vi "V7310.Job.Get.vi"(6 "timeout ms (5000)":i32=5000, 8 "error in":errorcluster, 11 "Connection in":refnum<k5>) -> (0 "error out":errorcluster, 2 "Job":string, 3 "Connection out":refnum<k5>)   [LabVIEW 2016]
uses:
  LowLevel/V7310.Commands.ctl
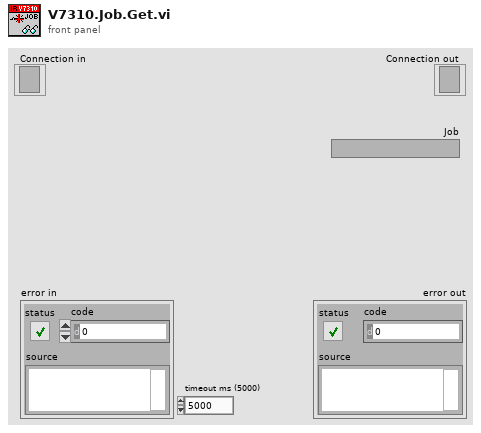
[diagram p1: front panel]
types:
  T1 = typedef "V7310.Commands.ctl" = enum16{"Start", "Stop", "GetStatus", "GetVarNames", "GetJobNames", "SetJob", "GetJob", "SetVars", "GetVars", "SetLayoutPosition", "SetRotation", "GetMessageID", "GetMessages", "ConfirmMessages", "DeleteMessages", "SetRTC", "GetRTC", "SetVarPosition", "SetIntensity", "GetIntensity", "SetStartTriggerDelay", "GetStartTriggerDelay", "SetStopTriggerDelay", "GetStopTriggerDelay", "SetConsecutiveTriggerDelay", "GetConsecutiveTriggerDelay", "SetMarkSpeed", "GetMarkSpeed"}
  T2 = typedef "V7310.ErrorLevels.ctl" = enum16{"OK", "Warning", "Error"}
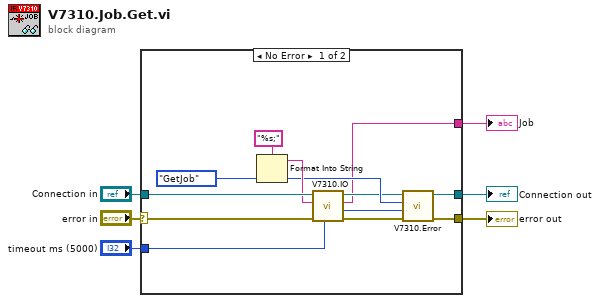
[diagram p0: block diagram]
diagram:
  n1 = case shown="No Error" "error in" {
    selector: "error in" -> [w16 w18]
    tunnel: "Connection in" -> [w17 w19]
    tunnel: [w8 w19] -> w5
    tunnel: "timeout ms (5000)" -> [w10 _]
    tunnel: [w9 w18] -> w2
    tunnel: [w7 _] -> w1
    frame No Error {
      w13 = V7310.Commands."GetJob" ("Cmd")
      n2 = Format Into String(format string="%s;", w13) -> (resulting string=w14:string)  [unwired: 2 in, 1 out]
      n3 = call "V7310.IO.vi"("timeout ms (5000)"=w10, "error in"=w16, "Data in"=w14, "Connection in"=w17) -> ("error out"=w11:errorcluster, "Error Level"=w12:T2, "Data out"=w7:string, "Connection out"=w8:refnum<k5>)  [unwired: 4 in]
      n4 = call "V7310.Error.vi"("error in"=w11, "Error Level"=w12, "Cmd"=w13) -> ("error out"=w9:errorcluster)  [unwired: 8 in]
    }
    frame Error {
    }
  }
  "Connection out" <- w5
  "error out" <- w2
  "Job" <- w1
